vi "z_control.vi"() -> ()   [LabVIEW 2017]
uses:
  controls/state_machine_TYPE.ctl
  <vilib>/Platform/TimedLoop/XDataNode/timing_clust.ctl
  <vilib>/Platform/TimedLoop/XDataNode/nitl_modes.ctl
  <vilib>/Platform/TimedLoop/XDataNode/wakeup.ctl
  <vilib>/rvi/IPIntegrationNode/IPINode_Typedef/niFpgaIPINodeSupportedFamilies.ctl
  <vilib>/rvi/Emulation/niFpgaSctlEmulationGetInTimedLoop.vi
  <vilib>/rvi/Emulation/niFpgaEmulationReportErrorSimple.vi
  <vilib>/rvi/Emulation/niFpgaGetClockAttributes.vi
  <vilib>/rvi/Emulation/niFpgaCriticalErrorInLSC.vi
  <vilib>/rvi/IPIntegrationNode/IPINode_Utilities/niFpgaIPINodeSimCore.vi
  <vilib>/platform/TimedLoop/XDataNode/XDataNode.xnode
  <vilib>/rvi/IPIntegrationNode/IPINode_Xnode/niFpgaIPINode.xnode
  Z_dash_controlSimFiles/z-control_569670B881CD4E418A5B0FD764EA802B.dll
  <vilib>/Platform/TimedLoop/XDataNode/XDNodeRunTimeDep.lvlib
panel:
  in  "Boolean array 2":bool[](array[boolean])=[FALSE, FALSE, FALSE, FALSE, FALSE, FALSE, FALSE, FALSE, FALSE, FALSE, FALSE, FALSE, FALSE, FALSE, FALSE, FALSE]
  out "r_slow 2":fxp<+/-,16,1>
  out "Boolean array":bool[](array[boolean])
  in  "Boolean 2":bool
  in  "r_slow":fxp<+/-,16,1>
  in  "r_fast":fxp<+/-,16,1>
  out "u_k":fxp<+,16,5>
  in  "fast_thresh":fxp<+/-,16,5>
  in  "u(k-1)":fxp<+/-,16,5>
  in  "state":T1
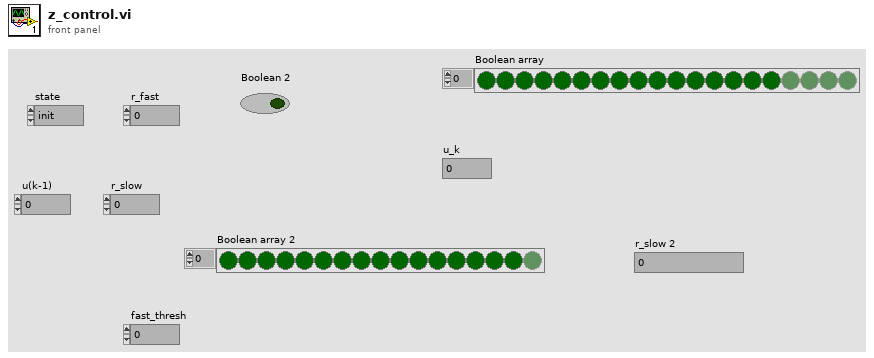
[diagram p1: front panel]
types:
  T1 = typedef "state_machine_TYPE.ctl" = enum16{"init", "xy", "z_eng", "z_settle", "measure", "z_up", ""}
  T2 = typedef "XDNodeRunTimeDep.lvlib/timing_clust.ctl" = cluster{"Expected End [f-1]":u64, "Actual End [f-1]":u64, "Finished Late? [f-1]":bool, "Expected End [i-1]":u64, "Actual End [i-1]":u64, "Finished Late? [i-1]":bool, "Expected Start [i]":u64, "Actual Start [i]":u64, "Expected Start [f]":u64, "Actual Start [f]":u64, "Source Name":string, "Structure Name":string, "Period":i64, "Deadline":i64, "Offset":i64, "Start":i64, "Priority":i32, "Timeout":i32, "Mode":T3, "Wakeup Reason":T4, "Error":errorcluster, "Source Type":string, "Secondary Source Type":string, "Global End Time":u64, "Global Start Time":u64, "Frame Duration":u64, "Iteration Duration":u64, "Assigned CPU":i32, "I/O Scan Engine Mode":u32}
  T3 = typedef "XDNodeRunTimeDep.lvlib/nitl_modes.ctl" = enum32{"No Change", "Process missed periods, maintain original phase", "Discard missed periods, maintain original phase", "Process missed periods, ignore original phase", "Discard missed periods, ignore original phase"}
  T4 = typedef "XDNodeRunTimeDep.lvlib/wakeup.ctl" = enum32{"Normal", "Aborted", "Asynchronous wakeup", "Timing source error", "Timed loop error", "Timeout"}
  T5 = typedef "niFpgaIPINodeSupportedFamilies.ctl" = cluster{"unlimited?":bool, "supported targets":string[]}
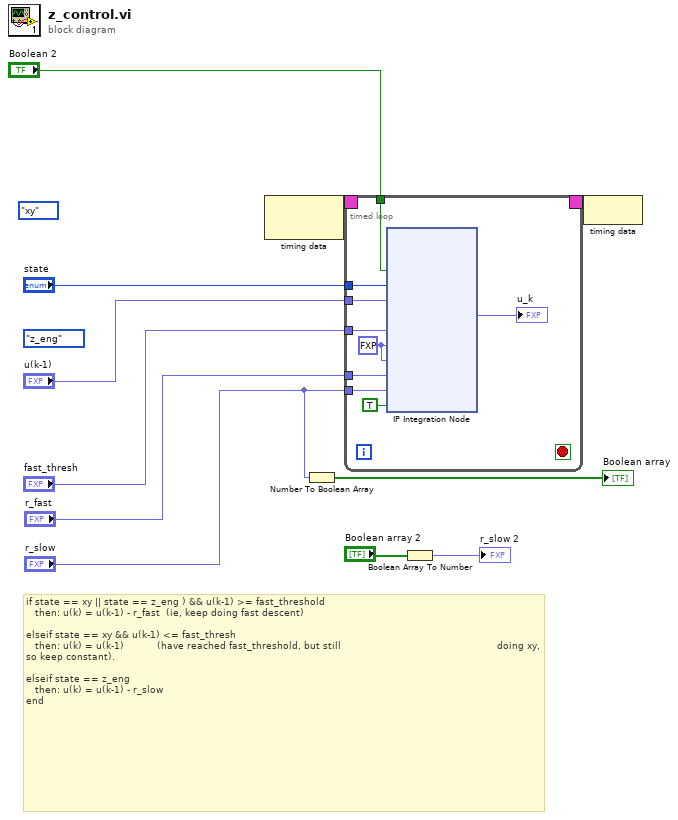
[diagram p0: block diagram]
diagram:
  (unwired) state_machine_TYPE."z_eng"
  (unwired) state_machine_TYPE."xy"
  # "if state == xy || state == z_eng ) && u(k-1) >= fast_threshold\n   then: u(k) = u(k-1) - r_fast  (ie, keep doing fast descent)\n\nelseif state == xy && u(k-1) <= fast_thresh\n   then: u(k) = u(k-1)           (have reached fast_threshold, but still                                                    doing xy, so keep constant).\n\nelseif state == z_eng\n   then: u(k) = u(k-1) - r_slow\nend"
  n1 = node-c288() -> (w2:T2)  [unwired: 1 in]
  n2 = Number To Boolean Array(number="r_slow") -> (Boolean array=→"Boolean array":bool[])
  n3 = timed-loop {
    timing: w2 -> [_]
    timing-out: [_] -> w1
    tunnel: "state" -> [w20]
    tunnel: "u(k-1)" -> [w19]
    tunnel: "fast_thresh" -> [w18]
    tunnel: "r_fast" -> [w16]
    tunnel: "r_slow" -> [w15]
    tunnel: "Boolean 2" -> [w14]
    stop <- _ stop-if-true
    w17 = fxp<+/-,16,5> 0.0 ("z_err")
    n4 = xnode "IP Integration Node"("sclr"=w14, "state"=w20, "u_kmin1"=w19, "fast_thresh"=w18, "z_err"=w17, "k_i"=w17, "r_fast"=w16, "r_slow"=w15, "ce"=TRUE) -> ("u_k"=→"u_k":fxp<+/-,16,5>)
  }
  n5 = Boolean Array To Number(Boolean array="Boolean array 2") -> (number=→"r_slow 2":fxp<+/-,16,1>)
  n6 = node-c288(w1) -> ()
